vi "ois_ttc_merging_v2.vi"() -> ()   [LabVIEW 2012]
uses:
  <vilib>/vision/Image Controls.llb/IMAQ Image.ctl
  <vilib>/vision/NI_Vision_Development_Module.lvlib
  <vilib>/Utility/file.llb/Write To Spreadsheet File (I64).vi
panel:
  in  "Tab Control":T1(tab)
  in  "save mask":bool
  in  "OIS file path":path=path "\\\\IFMB-02-024B-10\\Ischemia2/OOS/2019-05-27/2019-05-27_15-19-23.oos"
  out "IM":T2(plugin-control)
  out "mask":T2(plugin-control)
  out "marks":T2(plugin-control)
  in  "center Y":u32(slide)=123
  in  "center X":u32(slide)=241 scale=0.0..515.0
  in  "TTC Angle":dbl(knob)=360.0 caption="Angle"
  out "front TTC image":T2(plugin-control) caption="TTC image"
  in  "TTC Zoom":dbl(slide)=0.45869162995594714 caption="Zoom" scale=0.001..1.0
  in  "TTC vert reverse":bool caption="Vertical reverse"
  in  "TTC horiz reverse":bool caption="Horizontal reverse"
  in  "TTC image file path":path=path "\\\\ED02\\Data_Marat/Ischemia/TTC Elvira/270519_P8/slice1.tif"
  in  "save masked TTC":bool
  in  "Protocol folder":path=path "D:/Neurolab/Data/Ischemia/Traces/TTC_masked"
  in  "default TTC masked image save folder":path=path "D:/Neurolab/Data/Ischemia/Traces/TTC_masked"
  in  "IM line color":u32(colorbox)=16860
  in  "IM line Width":u32=2
  in  "marks line Width":u32=2
  in  "marks line color":u32(colorbox)=16711680
  in  "TTC divide coef":i32=5
  in  "error in":errorcluster
  out "error out":errorcluster
  out "TTC image in":T2
  out "OIS Image in":T2
  out "OIS Image resolution":i32[](array[numeric])=[348, 260]
  in  "default OIS mask save folder":path=path "D:/Neurolab/Data/Ischemia/Traces/OIS_mask"
  in  "stop":bool=TRUE
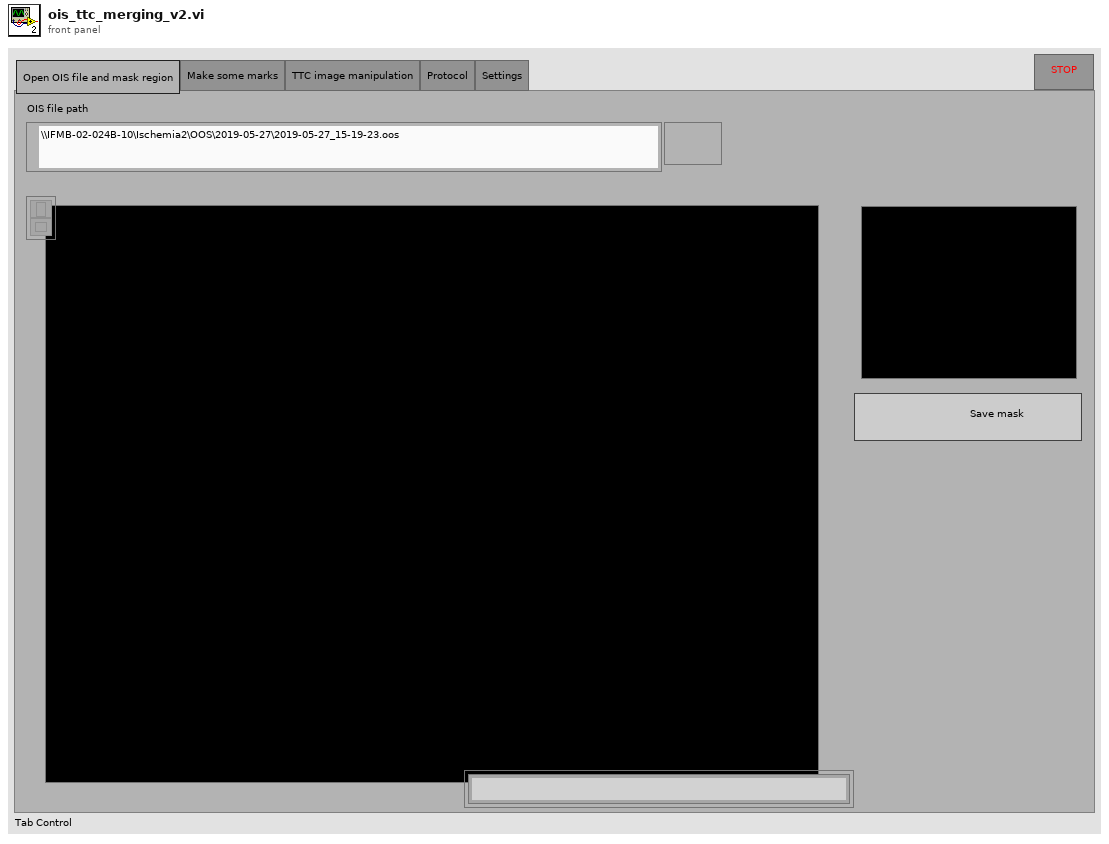
[diagram p1: front panel]
types:
  T1 = enum32{"Open OIS file and mask region", "Make some marks", "TTC image manipulation", "Protocol", "Settings"}
  T2 = typedef "IMAQ Image.ctl" = refnum<image>
  T3 = cluster{"Global Rectangle":i32[], "Contours":cluster{"Contour Type":u32, "ROI Type":u32, "Points":i32[]}[]}
  T4 = typedef "Image Type" = u32
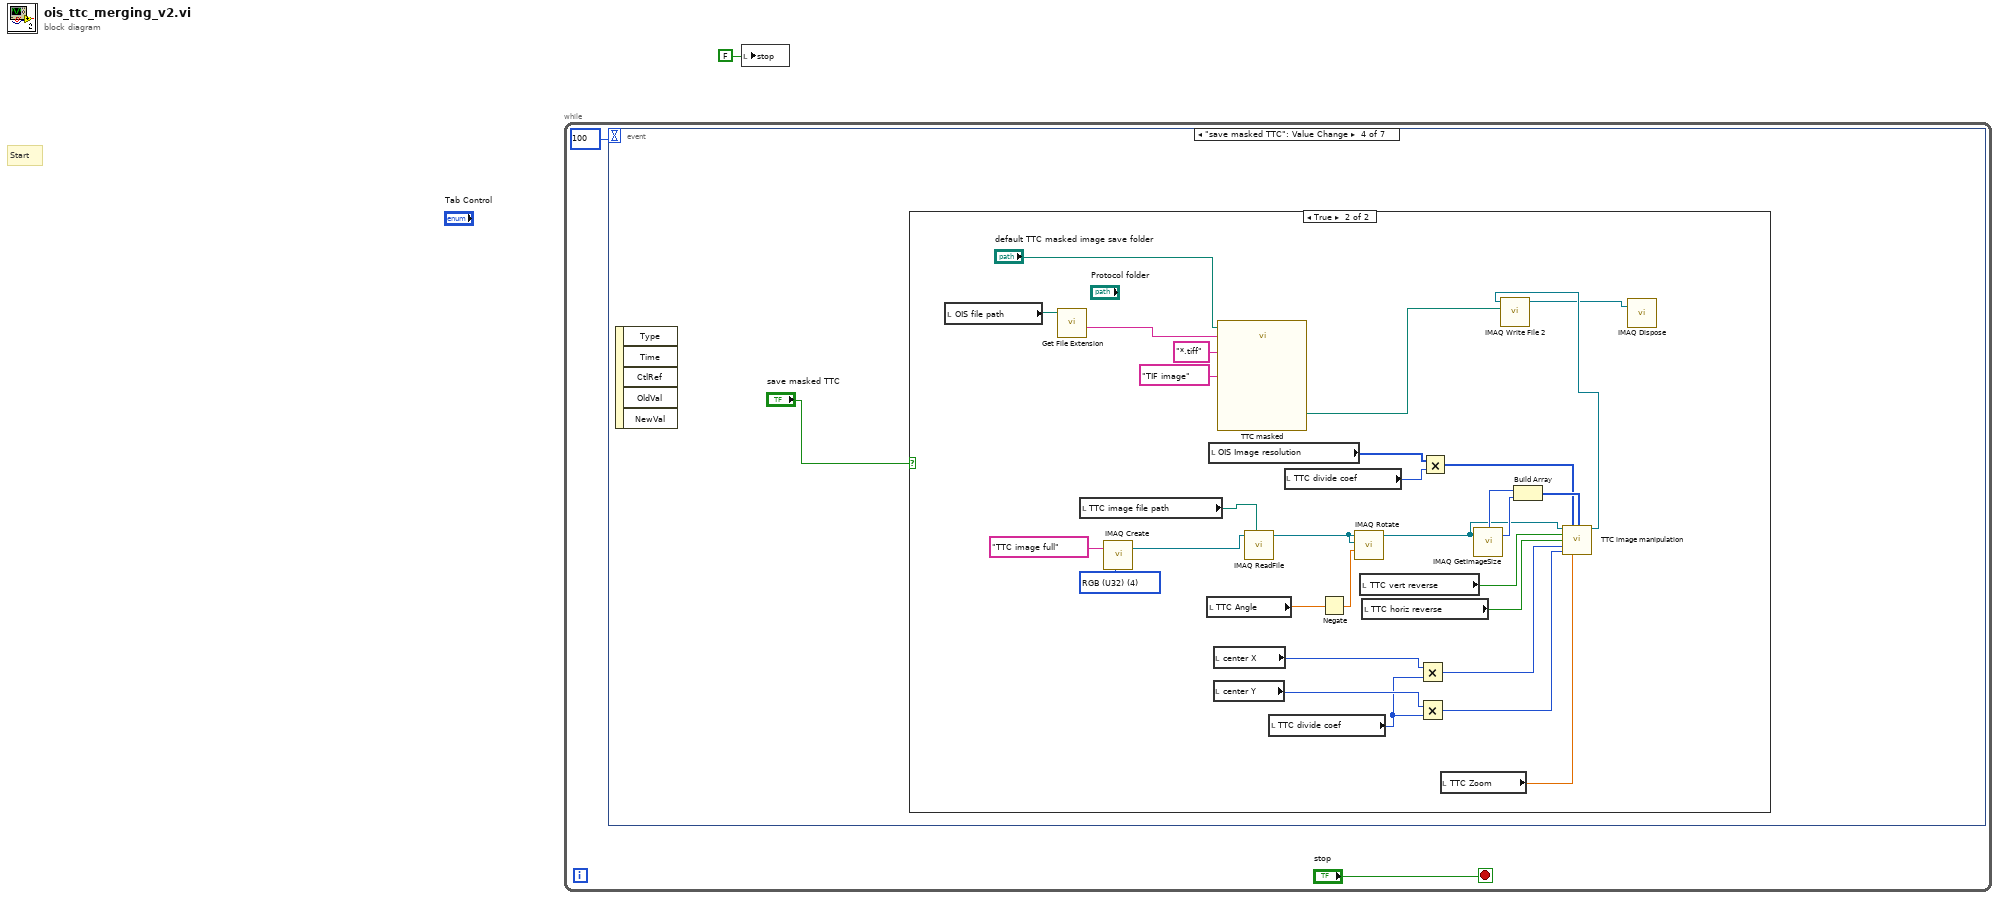
[diagram p0: block diagram]
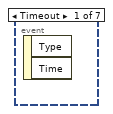
[diagram p2: hidden frame]
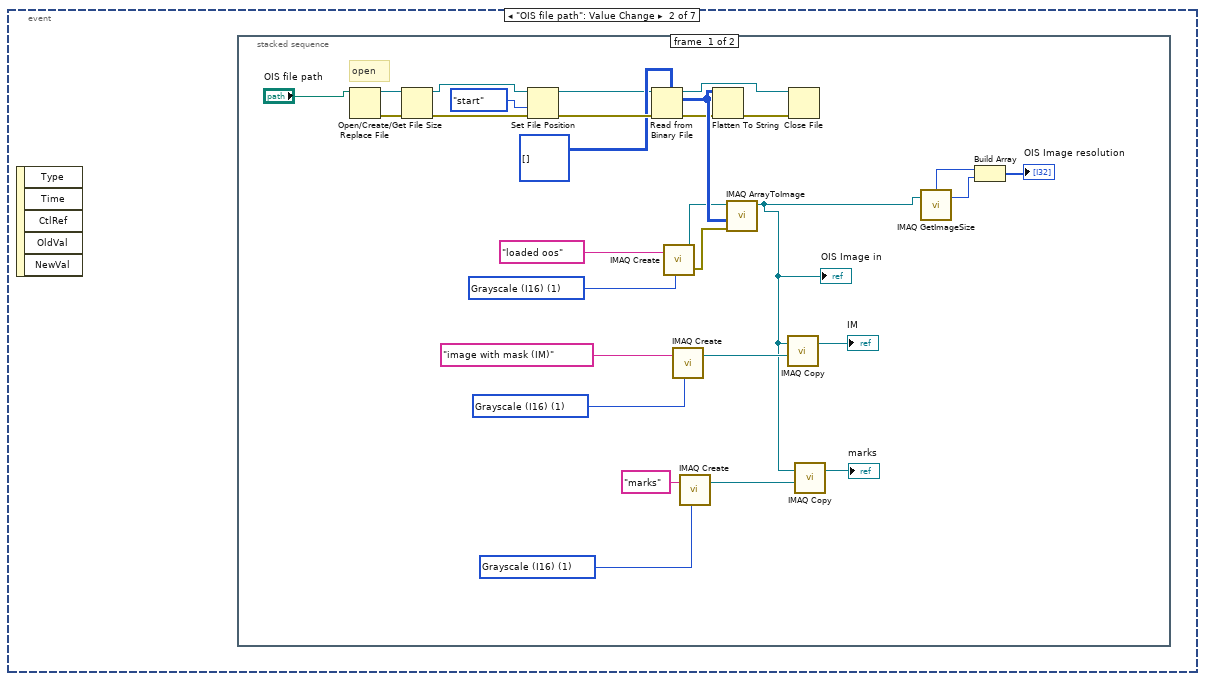
[diagram p3: hidden frame]
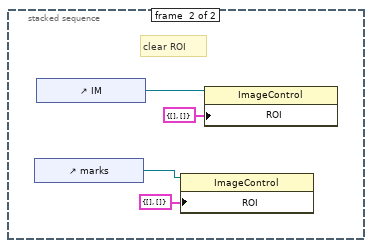
[diagram p4: hidden frame]
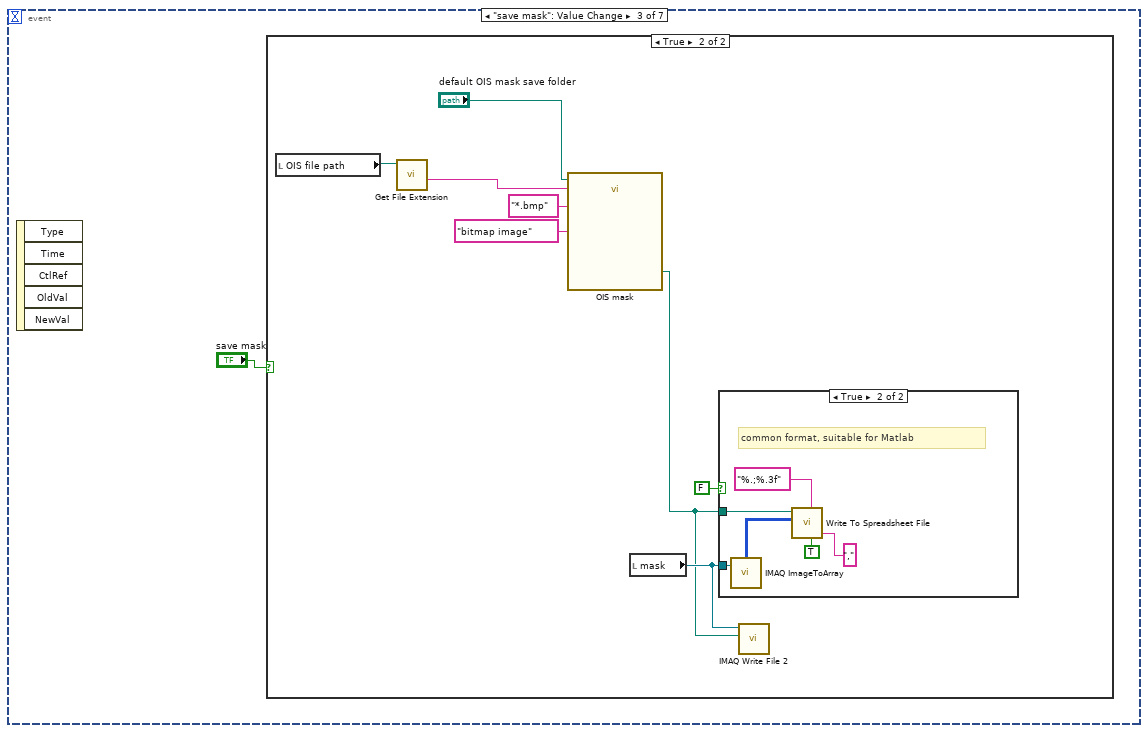
[diagram p5: hidden frame]
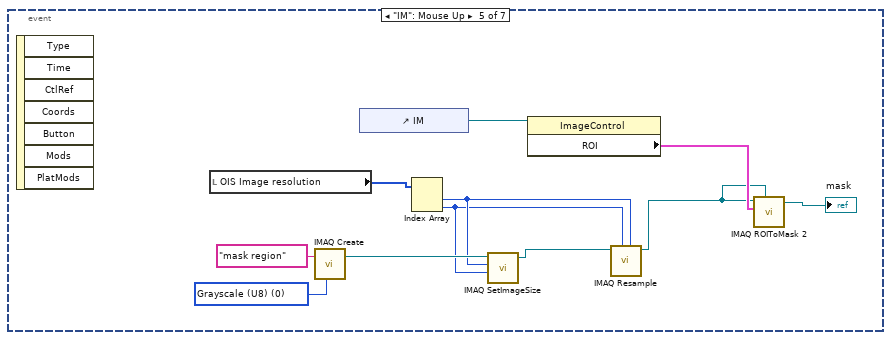
[diagram p9: hidden frame]
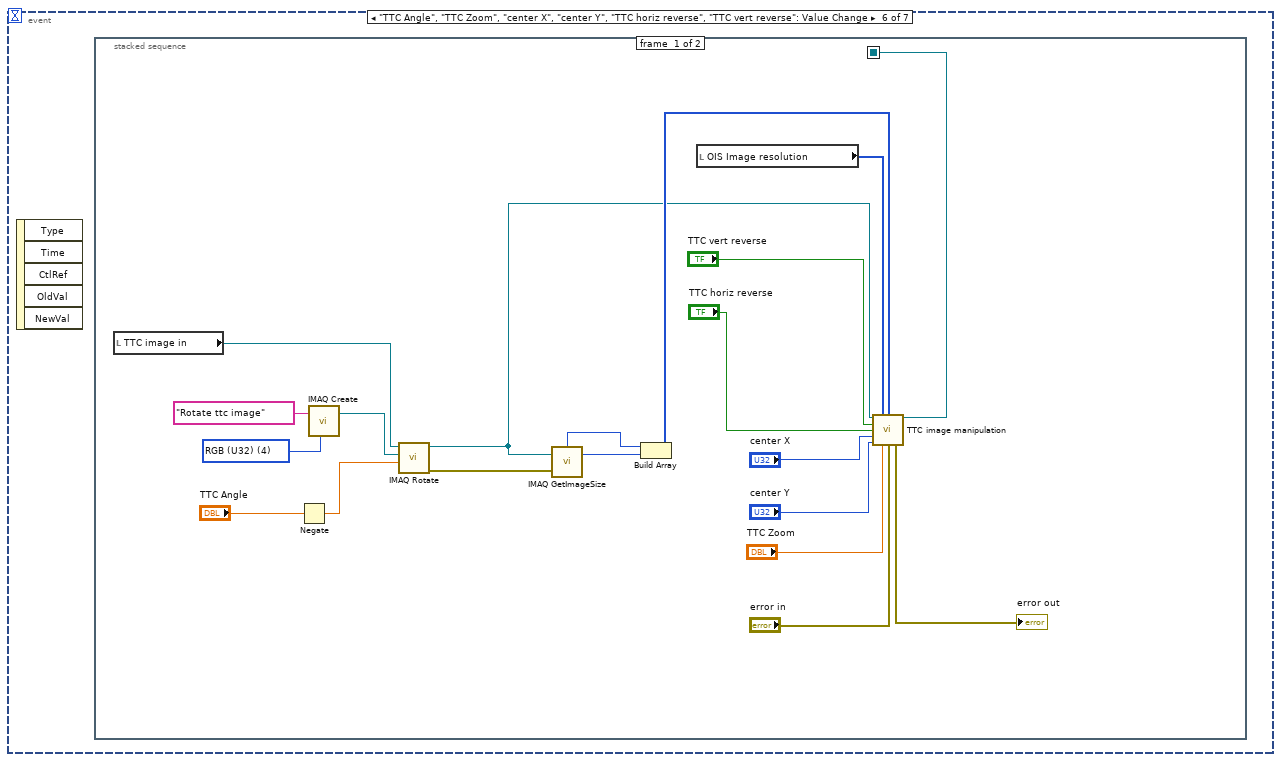
[diagram p10: hidden frame]
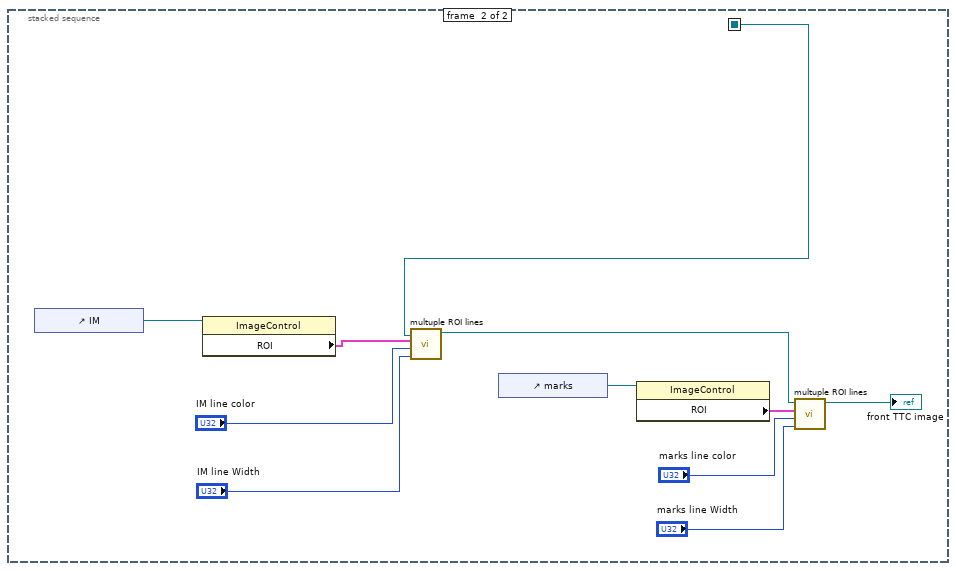
[diagram p11: hidden frame]
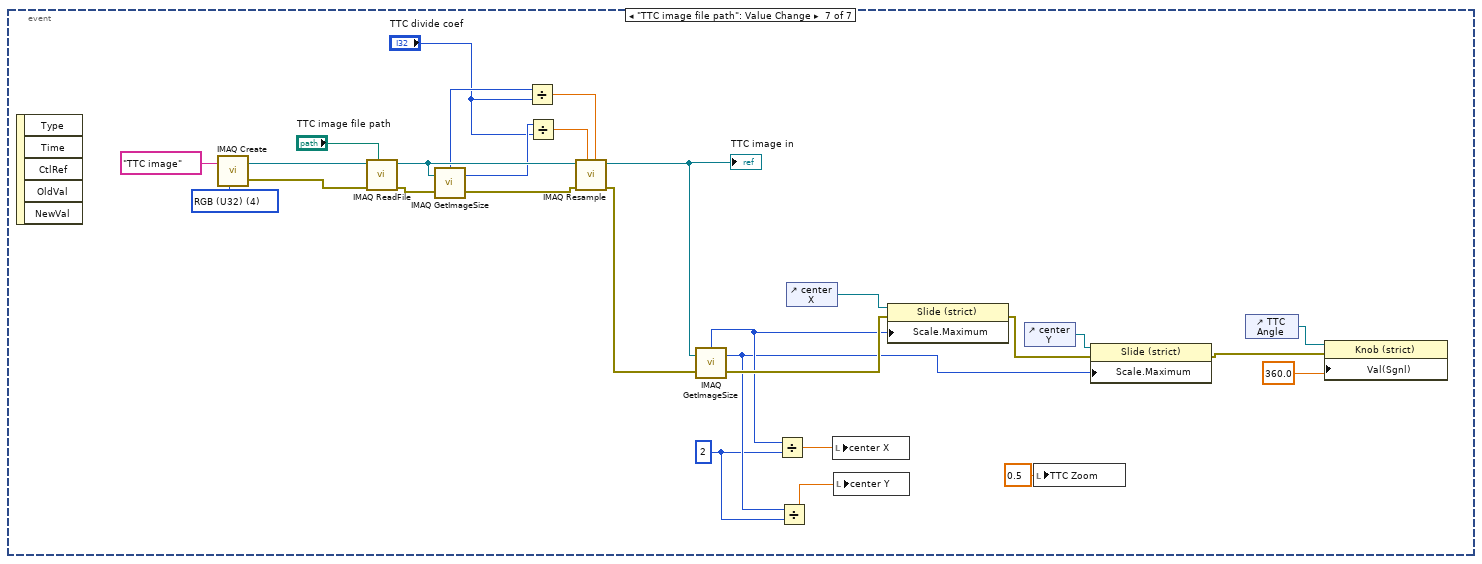
[diagram p12: hidden frame]
diagram:
  # "Start"
  n1 = while {
    stop <- "stop" stop-if-true
    n2 = event shown="[3] \"save masked TTC\": Value Change" {
      selector: _ -> [_ _ _ _ _ _ _]
      dyn-events: _ -> [_ _ _ _ _ _ _]
      timeout: 100 -> [_ _ _ _ _ _ _]
      event Timeout {
        n3 = event-data() -> ()  [unwired: 1 in, 2 out]
      }
      event "OIS file path": Value Change {
        n4 = event-data() -> ()  [unwired: 1 in, 5 out]
        n5 = stacked-sequence {
          frame #0 {
            w10 = T4 1 items=["Grayscale (U8)", "Grayscale (I16)", "Grayscale (SGL)", "Complex (CSG)", "RGB (U32)", "HSL (U32)", "RGB (U64)", "Grayscale (U16)"] ("Image Type")
            w14 = T4 1 items=["Grayscale (U8)", "Grayscale (I16)", "Grayscale (SGL)", "Complex (CSG)", "RGB (U32)", "HSL (U32)", "RGB (U64)", "Grayscale (U16)"] ("Image Type")
            w28 = T4 1 items=["Grayscale (U8)", "Grayscale (I16)", "Grayscale (SGL)", "Complex (CSG)", "RGB (U32)", "HSL (U32)", "RGB (U64)", "Grayscale (U16)"] ("Image Type")
            # "open"
            n6 = Open/Create/Replace File(file path (use dialog)="OIS file path") -> (refnum out=w16:refnum<file>, error out=w17:errorcluster)  [unwired: 5 in, 1 out]
            n7 = Get File Size(file=w16, error in=w17) -> (refnum out=w19:refnum<file>, 0:w24:errorcluster)  [unwired: 1 out]
            n8 = Set File Position(refnum=w19, from (0:start)=enum16{"start", "end", "current"}."start", error in=w24) -> (refnum out=w20:refnum<file>, error out=w25:errorcluster)  [unwired: 1 in]
            n9 = Read from Binary File(5:i16[][] [] ("Image Pixels (I16)"), 8:w25, 11:w20) -> (0:w21:errorcluster, 2:w32:i16[][], 3:w22:refnum<file>)  [unwired: 3 in, 1 out]
            n10 = call "IMAQ Create"("Image Name"="loaded oos", "Image Type"=w28) -> ("New Image"=w31:T2, "error out"=w30:errorcluster)  [unwired: 3 in]
            n11 = call "IMAQ Create"("Image Name"="image with mask (IM)", "Image Type"=w14) -> ("New Image"=w13:T2)  [unwired: 3 in, 1 out]
            n12 = call "IMAQ Create"("Image Name"="marks", "Image Type"=w10) -> ("New Image"=w11:T2)  [unwired: 3 in, 1 out]
            n13 = Flatten To String(anything=w32, error in (no error)=w21) -> (error out=w26:errorcluster)  [unwired: 2 in, 2 out]
            n14 = call "IMAQ ArrayToImage"("error in (no error)"=w30, "Image Pixels (I16)"=w32, "Image"=w31) -> ("Image Out"=w5:T2)  [unwired: 7 in, 1 out]
            "OIS Image in" <- w5
            n15 = call "IMAQ Copy"("Image Dst"=w13, "Image Src"=w5) -> ("Image Dst Out"=→"IM":T2)  [unwired: 4 in, 1 out]
            n16 = Close File(refnum=w22, error in=w26) -> ()  [unwired: 2 out]
            n17 = call "IMAQ Copy"("Image Dst"=w11, "Image Src"=w5) -> ("Image Dst Out"=→"marks":T2)  [unwired: 4 in, 1 out]
            n18 = call "IMAQ GetImageSize"("Image"=w5) -> ("Y Resolution"=w7:i32, "X Resolution"=w6:i32)  [unwired: 3 in, 1 out]
            n19 = Build Array(w6, w7) -> (→"OIS Image resolution":i32[])
          }
          frame #1 {
            # "clear ROI"
            n20 = control-ref of="marks"() -> (w34:refnum<vi>)
            n21 = control-ref of="IM"() -> (w36:refnum<vi>)
            n22 = property on="Property Node" class="ImageControl"(reference=w34, "ROI"=T3 {"Global Rectangle"=[], "Contours"=[]}) -> ()  [unwired: 1 in, 2 out]
            n23 = property on="Property Node" class="ImageControl"(reference=w36, "ROI"=T3 {"Global Rectangle"=[], "Contours"=[]}) -> ()  [unwired: 1 in, 2 out]
          }
        }
      }
      event "save mask": Value Change {
        n24 = event-data() -> ()  [unwired: 1 in, 5 out]
        n25 = case shown="True" "save mask" {
          frame False {
          }
          frame True {
            n26 = local read "OIS file path"() -> (w39:path)
            n27 = call <vilib>:"Get File Extension.vi"("file"=w39) -> ("filename without extension"=w38:string)  [unwired: 7 in, 3 out]
            n28 = call "OIS mask"("start path"="default OIS mask save folder", "default name"=w38, "pattern (all files)"="*.bmp", "pattern label"="bitmap image") -> ("selected path"=w40:path)  [unwired: 8 in, 3 out]
            n29 = local read "mask"() -> (w42:T2)
            n30 = case shown="True" FALSE {
              tunnel: w40 -> [_ w48]
              tunnel: w42 -> [_ w46]
              frame False {
              }
              frame True {
                # "common format, suitable for Matlab"
                n31 = call "IMAQ ImageToArray"("Image"=w46) -> ("Image Pixels (U8)"=w47:u8[][])  [unwired: 3 in, 4 out]
                n32 = call-poly <vilib>:"Write To Spreadsheet File.vi"("delimiter (\\t)"="," ("delimiter (\\t)"), "transpose? (no:F)"=TRUE, "format (%d)"="%.;%.3f" ("format (%.3f)"), "2D data"=w47, "file path (dialog if empty)"=w48) -> ()  [unwired: 3 in, 1 out]
              }
            }
            n33 = call-poly "IMAQ Write File 2"("File Path"=w40, "Image"=w42) -> ()  [unwired: 8 in, 2 out]
          }
        }
      }
      event "save masked TTC": Value Change {
        n34 = event-data() -> ()  [unwired: 1 in, 5 out]
        n35 = case shown="True" "save masked TTC" {
          frame False {
          }
          frame True {
            w72 = T4 4 items=["Grayscale (U8)", "Grayscale (I16)", "Grayscale (SGL)", "Complex (CSG)", "RGB (U32)", "HSL (U32)", "RGB (U64)", "Grayscale (U16)"] ("Image Type")
            n36 = local read "OIS file path"() -> (w80:path)
            n37 = call <vilib>:"Get File Extension.vi"("file"=w80) -> ("filename without extension"=w79:string)  [unwired: 7 in, 3 out]
            n38 = local read "TTC image file path"() -> (w75:path)
            n39 = call "IMAQ Create"("Image Name"="TTC image full", "Image Type"=w72) -> ("New Image"=w74:T2)  [unwired: 3 in, 1 out]
            n40 = local read "TTC Angle"() -> (w71:dbl)
            n41 = local read "OIS Image resolution"() -> (w61:i32[])
            n42 = local read "center X"() -> (w58:u32)
            n43 = local read "center Y"() -> (w57:u32)
            n44 = call "TTC masked"("start path"="default TTC masked image save folder", "default name"=w79, "pattern (all files)"="*.tiff", "pattern label"="TIF image") -> ("selected path"=w70:path)  [unwired: 8 in, 3 out]
            n45 = call "IMAQ ReadFile"("File Path"=w75, "Image"=w74) -> ("Image Out"=w76:T2)  [unwired: 5 in, 4 out]
            n46 = local read "TTC divide coef"() -> (w56:i32)
            n47 = local read "TTC divide coef"() -> (w60:i32)
            n48 = Negate(x=w71) -> (-x=w77:dbl)
            n49 = call "IMAQ Rotate"("Angle (degrees)"=w77, "Image Dst"=w76, "Image Src"=w76) -> ("Image Dst Out"=w63:T2)  [unwired: 7 in, 1 out]
            n50 = local read "TTC vert reverse"() -> (w64:bool)
            n51 = local read "TTC horiz reverse"() -> (w65:bool)
            n52 = Multiply(x=w58, y=w56) -> (x*y=w54:u32)
            n53 = Multiply(x=w57, y=w56) -> (x*y=w55:u32)
            n54 = Multiply(x=w61, y=w60) -> (x*y=w59:i32[])
            n55 = local read "TTC Zoom"() -> (w66:dbl)
            n56 = call "IMAQ GetImageSize"("Image"=w63) -> ("Y Resolution"=w68:i32, "X Resolution"=w69:i32)  [unwired: 3 in, 1 out]
            n57 = Build Array(w69, w68) -> (w67:i32[])
            n58 = call "TTC image manipulation.vi"("Image in"=w63, "OIS image resolution"=w59, "TTC image resolution"=w67, "TTC vertical reverse"=w64, "TTC horizontal reverse"=w65, "center X"=w54, "center Y"=w55, "TTC Zoom"=w66) -> ("Image out"=w62:T2)  [unwired: 4 in, 3 out]
            n59 = call-poly "IMAQ Write File 2"("File Path"=w70, "Image"=w62) -> ("Image Out (duplicate)"=w53:T2)  [unwired: 8 in, 1 out]
            n60 = call "IMAQ Dispose"("Image"=w53) -> ()  [unwired: 5 in, 1 out]
          }
        }
      }
      event "IM": Mouse Up {
        w92 = T4 0 items=["Grayscale (U8)", "Grayscale (I16)", "Grayscale (SGL)", "Complex (CSG)", "RGB (U32)", "HSL (U32)", "RGB (U64)", "Grayscale (U16)"] ("Image Type")
        n61 = event-data() -> ()  [unwired: 1 in, 7 out]
        n62 = local read "OIS Image resolution"() -> (w89:i32[])
        n63 = call "IMAQ Create"("Image Name"="mask region", "Image Type"=w92) -> ("New Image"=w88:T2)  [unwired: 3 in, 1 out]
        n64 = control-ref of="IM"() -> (w90:refnum<vi>)
        n65 = Index Array(array=w89) -> (element #1=w87:i32, element #2=w86:i32)  [unwired: 2 in]
        n66 = call "IMAQ SetImageSize"("Y Resolution"=w86, "X Resolution"=w87, "Image"=w88) -> ("Image Out"=w85:T2)  [unwired: 2 in, 1 out]
        n67 = property on="Property Node" class="ImageControl"(reference=w90) -> ("ROI"=w93:T3)  [unwired: 1 in, 2 out]
        n68 = call "IMAQ Resample"("X Resolution"=w87, "Y Resolution"=w86, "Image Src"=w85) -> ("Image Dst Out"=w84:T2)  [unwired: 7 in, 1 out]
        n69 = call "IMAQ ROIToMask 2"("Image Model"=w84, "ROI Descriptor"=w93, "Image"=w84) -> ("Image Out"=→"mask":T2)  [unwired: 6 in, 2 out]
      }
      event "TTC Angle", "TTC Zoom", "center X", "center Y", "TTC horiz reverse", "TTC vert reverse": Value Change {
        n70 = event-data() -> ()  [unwired: 1 in, 5 out]
        n71 = stacked-sequence {
          seq-local: [w99 _] -> [_ w115]
          frame #0 {
            w110 = T4 4 items=["Grayscale (U8)", "Grayscale (I16)", "Grayscale (SGL)", "Complex (CSG)", "RGB (U32)", "HSL (U32)", "RGB (U64)", "Grayscale (U16)"] ("Image Type")
            n72 = local read "TTC image in"() -> (w97:T2)
            n73 = Negate(x="TTC Angle") -> (-x=w96:dbl)
            n74 = call "IMAQ Create"("Image Name"="Rotate ttc image", "Image Type"=w110) -> ("New Image"=w109:T2)  [unwired: 3 in, 1 out]
            n75 = call "IMAQ Rotate"("Angle (degrees)"=w96, "Image Dst"=w109, "Image Src"=w97) -> ("error out"=w107:errorcluster, "Image Dst Out"=w98:T2)  [unwired: 7 in]
            n76 = call "IMAQ GetImageSize"("Image"=w98, "error in (no error)"=w107) -> ("Y Resolution"=w112:i32, "X Resolution"=w113:i32)  [unwired: 2 in, 1 out]
            n77 = Build Array(w113, w112) -> (w101:i32[])
            n78 = local read "OIS Image resolution"() -> (w100:i32[])
            n79 = call "TTC image manipulation.vi"("Image in"=w98, "OIS image resolution"=w100, "TTC image resolution"=w101, "TTC vertical reverse"="TTC vert reverse", "TTC horizontal reverse"="TTC horiz reverse", "center X"="center X", "center Y"="center Y", "TTC Zoom"="TTC Zoom", "error in (no error)"="error in") -> ("Image out"=w99:T2, "error out"=→"error out":errorcluster)  [unwired: 3 in, 2 out]
          }
          frame #1 {
            n80 = control-ref of="IM"() -> (w118:refnum<vi>)
            n81 = property on="Property Node" class="ImageControl"(reference=w118) -> ("ROI"=w114:T3)  [unwired: 1 in, 2 out]
            n82 = call "multuple ROI lines.vi"("Width"="IM line Width", "line color"="IM line color", "ROI"=w114, "Image in"=w115) -> ("Image out"=w123:T2)  [unwired: 7 in]
            n83 = control-ref of="marks"() -> (w119:refnum<vi>)
            n84 = property on="Property Node" class="ImageControl"(reference=w119) -> ("ROI"=w122:T3)  [unwired: 1 in, 2 out]
            n85 = call "multuple ROI lines.vi"("Width"="marks line Width", "line color"="marks line color", "ROI"=w122, "Image in"=w123) -> ("Image out"=→"front TTC image":T2)  [unwired: 7 in]
          }
        }
      }
      event "TTC image file path": Value Change {
        w126 = 2 ("y")
        w150 = T4 4 items=["Grayscale (U8)", "Grayscale (I16)", "Grayscale (SGL)", "Complex (CSG)", "RGB (U32)", "HSL (U32)", "RGB (U64)", "Grayscale (U16)"] ("Image Type")
        n86 = event-data() -> ()  [unwired: 1 in, 5 out]
        n87 = call "IMAQ Create"("Image Name"="TTC image", "Image Type"=w150) -> ("New Image"=w151:T2, "error out"=w148:errorcluster)  [unwired: 3 in]
        n88 = call "IMAQ ReadFile"("File Path"="TTC image file path", "error in (no error)"=w148, "Image"=w151) -> ("error out"=w133:errorcluster, "Image Out"=w140:T2)  [unwired: 4 in, 3 out]
        n89 = call "IMAQ GetImageSize"("Image"=w140, "error in (no error)"=w133) -> ("Y Resolution"=w138:i32, "X Resolution"=w139:i32, "error out"=w134:errorcluster)  [unwired: 2 in]
        n90 = Divide(x=w139, y="TTC divide coef") -> (x/y=w135:dbl)
        n91 = Divide(x=w138, y="TTC divide coef") -> (x/y=w136:dbl)
        n92 = call "IMAQ Resample"("X Resolution"=w135, "Y Resolution"=w136, "error in (no error)"=w134, "Image Src"=w140) -> ("error out"=w132:errorcluster, "Image Dst Out"=w131:T2)  [unwired: 6 in]
        "TTC image in" <- w131
        n93 = call "IMAQ GetImageSize"("Image"=w131, "error in (no error)"=w132) -> ("Y Resolution"=w127:i32, "X Resolution"=w130:i32, "error out"=w144:errorcluster)  [unwired: 2 in]
        n94 = Divide(x=w130, y=w126) -> (x/y=w129:dbl)
        n95 = Divide(x=w127, y=w126) -> (x/y=w128:dbl)
        n96 = control-ref of="center X"() -> (w147:refnum<vi>)
        n97 = local write "center X"(w129) -> ()
        n98 = local write "center Y"(w128) -> ()
        n99 = property on="Property Node" class="Slide (strict)"(reference=w147, error in=w144, "Scale.Maximum"=w130) -> (error out=w146:errorcluster)  [unwired: 1 out]
        n100 = control-ref of="center Y"() -> (w145:refnum<vi>)
        n101 = local write "TTC Zoom"(0.5 ("center X")) -> ()
        n102 = property on="Property Node" class="Slide (strict)"(reference=w145, error in=w146, "Scale.Maximum"=w127) -> (error out=w141:errorcluster)  [unwired: 1 out]
        n103 = control-ref of="TTC Angle"() -> (w142:refnum<vi>)
        n104 = property on="Property Node" class="Knob (strict)"(reference=w142, error in=w141, "Val(Sgnl)"=360.0 ("Value (Signaling)")) -> ()  [unwired: 2 out]
      }
    }
  }
  n105 = local write "stop"(FALSE ("stop")) -> ()
